vi "Ultra_Sonic.vi"(1 "output cluster 3":T1) -> (0 "Ultar_Sonic":T10)   [LabVIEW 2015]
uses:
  Ref_Num/DIO_Type_Def.ctl
  <vilib>/Rock Robotics/WPI/Ultrasonic/WPI_SonarMB1010DigitalDeviceRef.ctl
  <vilib>/Rock Robotics/WPI/Counter/WPI_CounterDevRef.ctl
  <vilib>/Rock Robotics/SystemInterfaces/Counter/FPGA_CounterCtrSystemIndex.ctl
  <vilib>/Rock Robotics/WPI/Encoder/WPI_EncoderDevRef.ctl
  <vilib>/Rock Robotics/SystemInterfaces/Encoder/FPGA_EncoderIdx.ctl
  <vilib>/Rock Robotics/WPI/Encoder/WPI_EncoderType.ctl
  <vilib>/Rock Robotics/WPI/DigitalInput/WPI_DigitalInputDevRef.ctl
  <vilib>/Rock Robotics/SystemInterfaces/DIO/FPGA_DIOChannel.ctl
  <vilib>/Rock Robotics/WPI/Ultrasonic/WPI_SonarMB1010DigitalGetRange.vi
panel:
  out "Waveform Chart":cluster{"Out":dbl, "Distance":dbl}(graph)
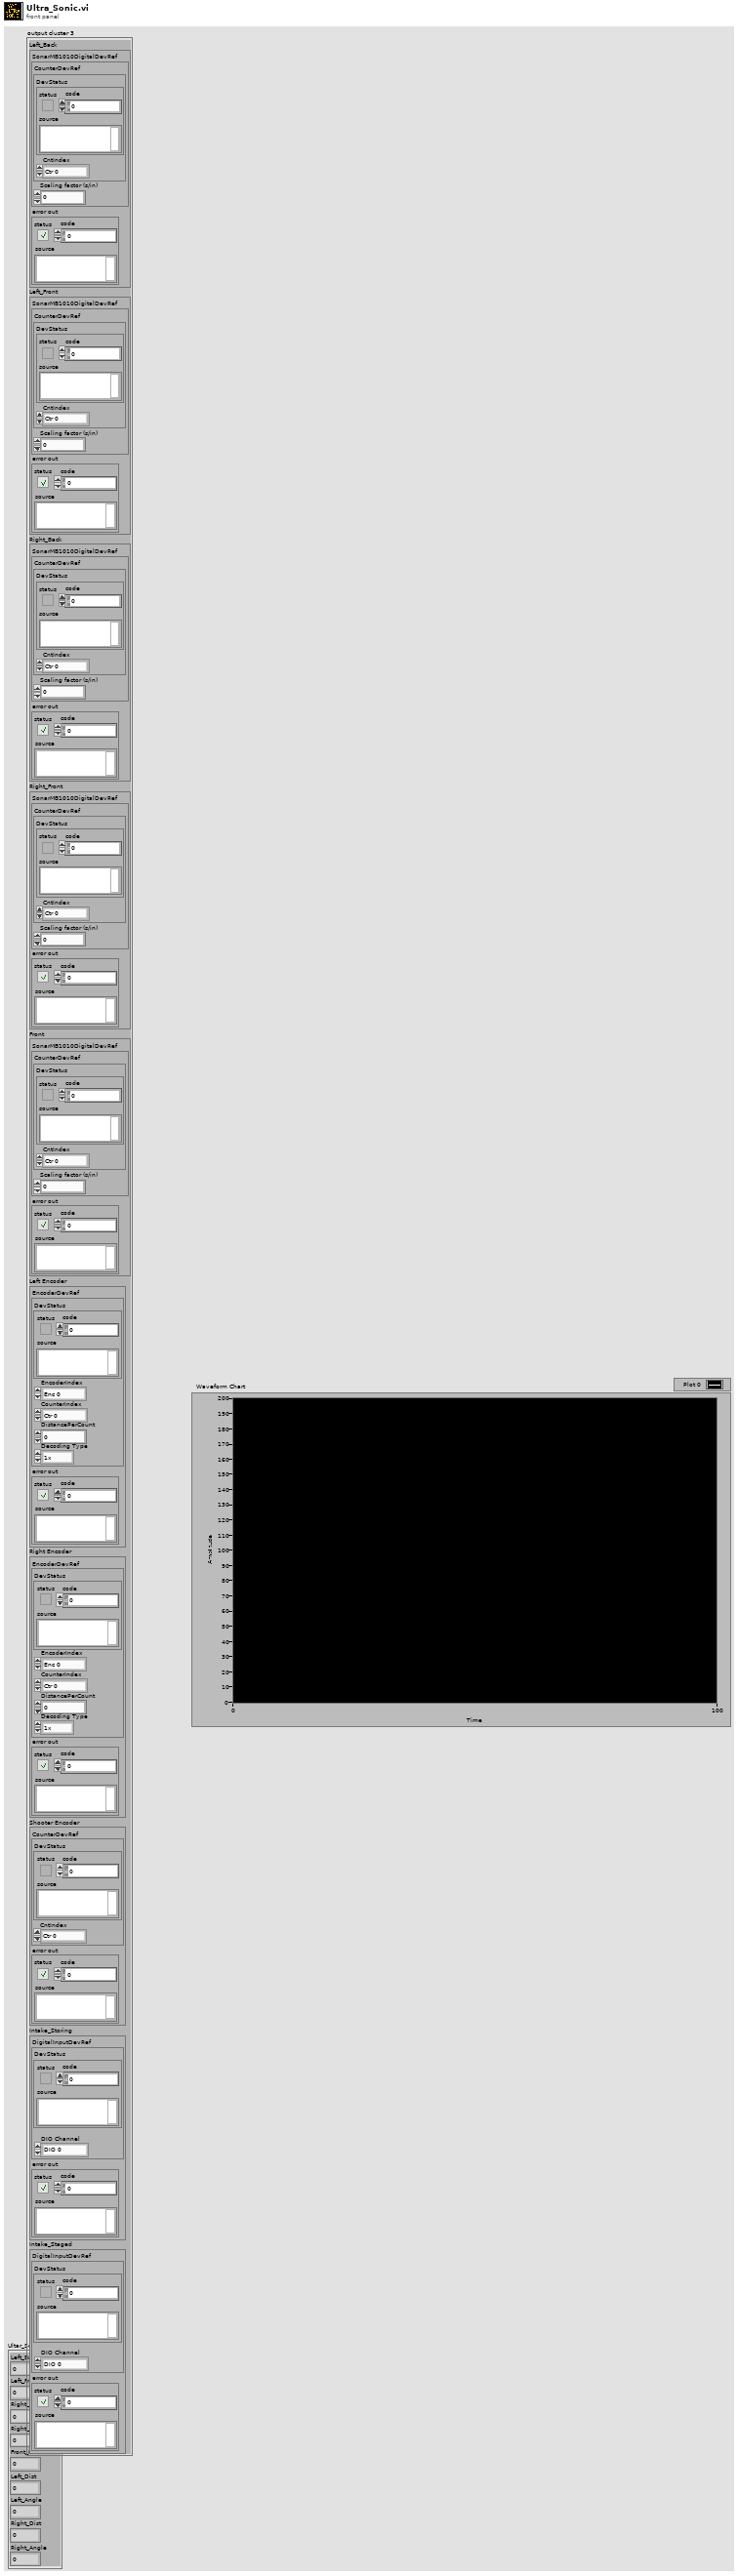
[diagram p1: front panel]
types:
  T1 = typedef "DIO_Type_Def.ctl" = cluster{"Left_Back":cluster{"SonarMB1010DigitalDevRef":T2, "error out":errorcluster}, "Left_Front":cluster{"SonarMB1010DigitalDevRef":T2, "error out":errorcluster}, "Right_Back":cluster{"SonarMB1010DigitalDevRef":T2, "error out":errorcluster}, "Right_Front":cluster{"SonarMB1010DigitalDevRef":T2, "error out":errorcluster}, "Front":cluster{"SonarMB1010DigitalDevRef":T2, "error out":errorcluster}, "Left Encoder":cluster{"EncoderDevRef":T5, "error out":errorcluster}, "Right Encoder":cluster{"EncoderDevRef":T5, "error out":errorcluster}, "Shooter Encoder":cluster{"CounterDevRef":T3, "error out":errorcluster}, "Intake_Storing":cluster{"DigitalInputDevRef":T8, "error out":errorcluster}, "Intake_Staged":cluster{"DigitalInputDevRef":T8, "error out":errorcluster}}
  T2 = typedef "WPI_SonarMB1010DigitalDeviceRef.ctl" = cluster{"CounterDevRef":T3, "Scaling factor (s/in)":dbl}
  T3 = typedef "WPI_CounterDevRef.ctl" = cluster{"DevStatus":errorcluster, "CntIndex":T4}
  T4 = typedef "FPGA_CounterCtrSystemIndex.ctl" = enum8{"Ctr 0", "Ctr 1", "Ctr 2", "Ctr 3", "Ctr 4", "Ctr 5", "Ctr 6", "Ctr 7", "Invalid"}
  T5 = typedef "WPI_EncoderDevRef.ctl" = cluster{"DevStatus":errorcluster, "EncoderIndex":T6, "CounterIndex":T4, "DistancePerCount":dbl, "Decoding Type":T7}
  T6 = typedef "FPGA_EncoderIdx.ctl" = enum8{"Enc 0", "Enc 1", "Enc 2", "Enc 3", "Enc 4", "Enc 5", "Enc 6", "Enc 7", "Invalid"}
  T7 = typedef "WPI_EncoderType.ctl" = enum16{"1x", "2x", "4x"}
  T8 = typedef "WPI_DigitalInputDevRef.ctl" = cluster{"DevStatus":errorcluster, "DIO Channel":T9}
  T9 = typedef "FPGA_DIOChannel.ctl" = enum8{"DIO 0", "DIO 1", "DIO 2", "DIO 3", "DIO 4", "DIO 5", "DIO 6", "DIO 7", "DIO 8", "DIO 9", "DIO MXP 0", "DIO MXP 1", "DIO MXP 2", "DIO MXP 3", "DIO MXP 4", "DIO MXP 5", "DIO MXP 6", "DIO MXP 7", "DIO MXP 8", "DIO MXP 9", "DIO MXP 10", "DIO MXP 11", "DIO MXP 12", "DIO MXP 13", "DIO MXP 14", "DIO MXP 15", "Invalid"}
  T10 = cluster{"Left_Back_Dist":dbl, "Left_Front_Dist":dbl, "Right_Back_Dist":dbl, "Right_Front_Dist":dbl, "Front_Dist":dbl, "Left_Dist":dbl, "Left_Angle":dbl, "Right_Dist":dbl, "Right_Angle":dbl}
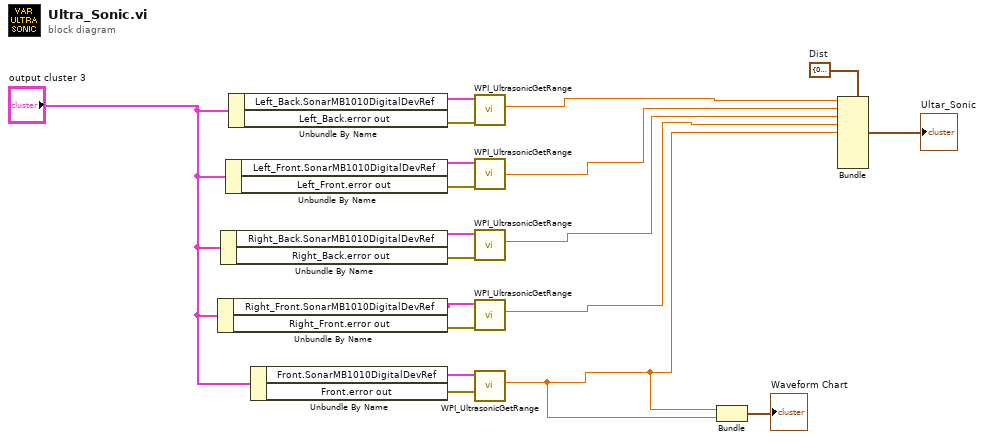
[diagram p0: block diagram]
diagram:
  w9 = T10 {"Left_Back_Dist"=0.0, "Left_Front_Dist"=0.0, "Right_Back_Dist"=0.0, "Right_Front_Dist"=0.0, "Front_Dist"=0.0, "Left_Dist"=0.0, "Left_Angle"=0.0, "Right_Dist"=0.0, "Right_Angle"=0.0}  # Dist
  n1 = Unbundle By Name("output cluster 3") -> ("Right_Front.SonarMB1010DigitalDevRef"=w13:T2, "Right_Front.error out"=w12:errorcluster)
  n2 = Unbundle By Name("output cluster 3") -> ("Right_Back.SonarMB1010DigitalDevRef"=w15:T2, "Right_Back.error out"=w14:errorcluster)
  n3 = Unbundle By Name("output cluster 3") -> ("Left_Front.SonarMB1010DigitalDevRef"=w17:T2, "Left_Front.error out"=w16:errorcluster)
  n4 = Unbundle By Name("output cluster 3") -> ("Left_Back.SonarMB1010DigitalDevRef"=w19:T2, "Left_Back.error out"=w18:errorcluster)
  n5 = Unbundle By Name("output cluster 3") -> ("Front.SonarMB1010DigitalDevRef"=w10:T2, "Front.error out"=w11:errorcluster)
  n6 = call-poly <vilib>:"WPI_UltrasonicGetRange.vi"("error in"=w18, "SonarMB1010DigitalDevRef"=w19) -> ("Distance"=w5:dbl)  [unwired: 7 in, 2 out]
  n7 = call-poly <vilib>:"WPI_UltrasonicGetRange.vi"("error in"=w16, "SonarMB1010DigitalDevRef"=w17) -> ("Distance"=w4:dbl)  [unwired: 7 in, 2 out]
  n8 = call-poly <vilib>:"WPI_UltrasonicGetRange.vi"("error in"=w14, "SonarMB1010DigitalDevRef"=w15) -> ("Distance"=w3:dbl)  [unwired: 7 in, 2 out]
  n9 = call-poly <vilib>:"WPI_UltrasonicGetRange.vi"("error in"=w12, "SonarMB1010DigitalDevRef"=w13) -> ("Distance"=w2:dbl)  [unwired: 7 in, 2 out]
  n10 = call-poly <vilib>:"WPI_UltrasonicGetRange.vi"("error in"=w11, "SonarMB1010DigitalDevRef"=w10) -> ("Distance"=w1:dbl)  [unwired: 7 in, 2 out]
  n11 = Bundle("Distance"=w1, "Distance"=w1) -> (→"Waveform Chart":cluster{"Distance":dbl, "Distance":dbl})  [unwired: 1 in]
  n12 = Bundle(cluster=w9, "Left_Back_Dist"=w5, "Left_Front_Dist"=w4, "Right_Back_Dist"=w3, "Right_Front_Dist"=w2, "Front_Dist"=w1) -> (→"Ultar_Sonic":T10)  [unwired: 4 in]
